vi "Turn.vi"(5 "角度":dbl format="%#_13g", 11 "error in (no error)":errorcluster) -> (15 "error out":errorcluster)   [LabVIEW 2019]
panel:
  out "馬達電壓":dbl[][](graph)
  out "SPD":dbl[](graph)
  out "POS":dbl[](graph)
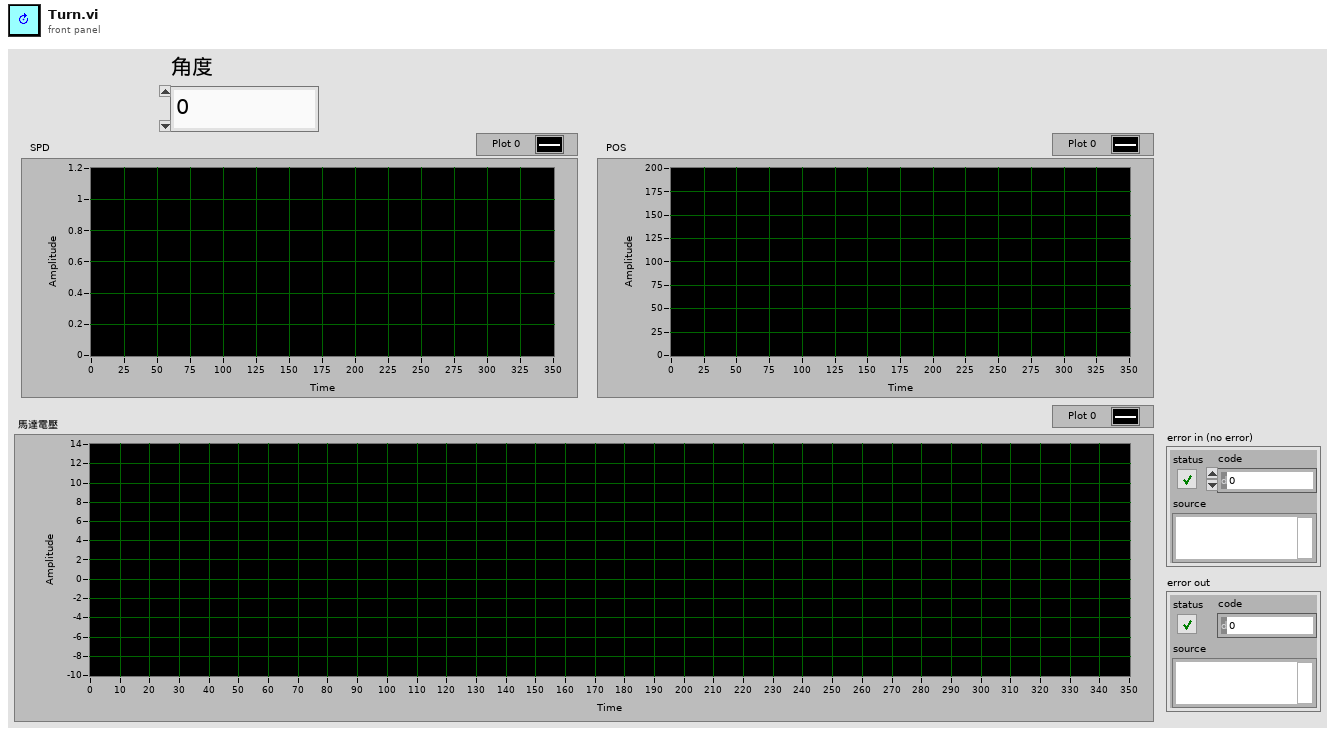
[diagram p1: front panel]
types:
  T1 = cluster{"proportional gain (Kc)":dbl, "integral time (Ti, min)":dbl, "derivative time (Td, min)":dbl}
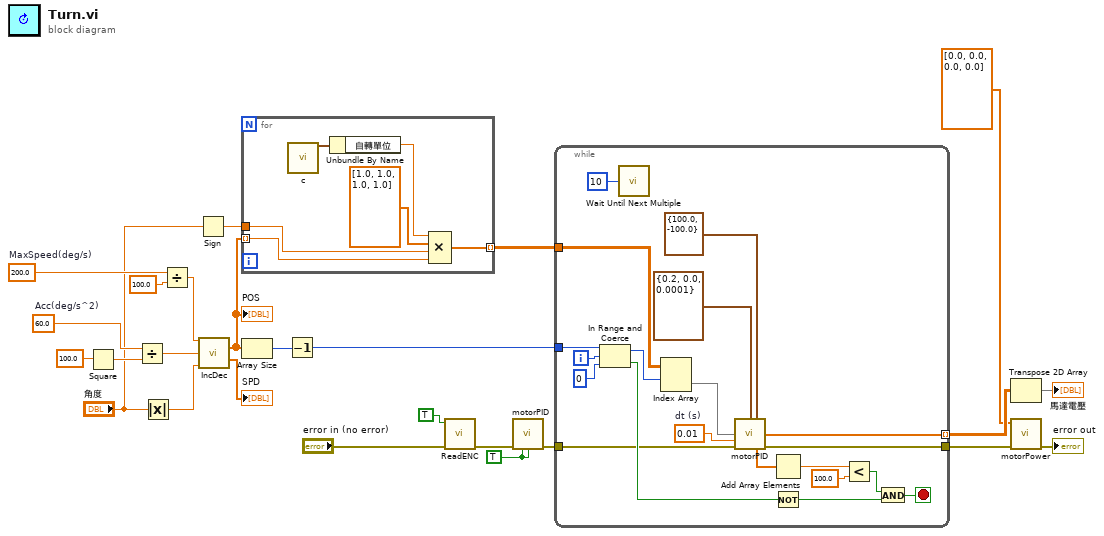
[diagram p0: block diagram]
diagram:
  w7 = 60.0  # Acc(deg/s^2)
  w4 = 200.0  # MaxSpeed(deg/s)
  w19 = TRUE ("reinitialize? (F)")
  n1 = Square(x=100.0 ("y")) -> (x^2=w14:dbl)
  n2 = Divide(x=w7, y=w14) -> (x/y=w15:dbl)
  n3 = Absolute Value(x="角度") -> (abs(x)=w11:dbl)
  n4 = Divide(x=w4, y=100.0) -> (x/y=w10:dbl)
  n5 = Sign(1:"角度") -> (0:w9:dbl)
  n6 = call "IncDec.vi"("MaxSpeed"=w10, "Acc"=w15, "Target"=w11) -> ("Position"=w12:dbl[], "Speed"=→"SPD":dbl[])  [unwired: 11 in]
  "POS" <- w12
  n7 = for {
    tunnel: w12 -> [w29] mode=indexing
    tunnel: [w31] -> w1 mode=indexing
    tunnel: w9 -> [w28]
    n8 = call "c.vi"() -> ("移動單位"=w27:cluster{"移動單位":dbl, "自轉單位":dbl})  [unwired: 15 in]
    n9 = Unbundle By Name(w27) -> ("自轉單位"=w30:dbl)
    n10 = Compound Arithmetic op=MULTIPLY(w30, dbl[] [1.0, 1.0, 1.0, 1.0] ("y"), w28, w29) -> (w31:dbl[])
  }
  n11 = Array Size(array=w12) -> (size(s)=w8:i32)
  n12 = Decrement(x=w8) -> (x-1=w2:i32)
  n13 = call "ReadENC.vi"("error in (no error)"="error in (no error)", "Reset"=TRUE) -> ("error out"=w18:errorcluster)  [unwired: 8 in, 1 out]
  n14 = call "motorPID.vi"("error in (no error)"=w18, "reinitialize? (F)"=w19, "EncRst"=w19) -> ("error out"=w20:errorcluster)  [unwired: 9 in, 3 out]
  n15 = while {
    tunnel: [w37] -> w25 mode=indexing
    tunnel: w20 -> [w35]
    tunnel: [w34] -> w22
    tunnel: w2 -> [w33]
    tunnel: w1 -> [w32]
    i -> [w43]
    stop <- w42 stop-if-true
    w38 = 0.01  # dt (s)
    n16 = In Range and Coerce(upper limit=w33, x=w43, lower limit=0) -> (coerced(x)=w47:i32, In Range?=w46:bool)
    n17 = call "Wait Until Next Multiple"("Count(mSec)"=u32 10) -> ()  [unwired: 1 out]
    n18 = Index Array(array=w32, index (row)=w47) -> (element=w39:dbl[])  [unwired: 1 in]
    n19 = call "motorPID.vi"("PID gains"=T1 {"proportional gain (Kc)"=0.2, "integral time (Ti, min)"=0.0, "derivative time (Td, min)"=0.0001}, "output range"=cluster{"output high":dbl, "output low":dbl} {"output high"=100.0, "output low"=-100.0}, "目標"=w39, "dt (s)"=w38, "error in (no error)"=w35) -> ("power"=w37:dbl[], "差值"=w36:dbl[], "error out"=w34:errorcluster)  [unwired: 7 in, 1 out]
    n20 = Add Array Elements(numeric array=w36) -> (sum=w50:dbl)
    n21 = Not(x=w46) -> (.not. x?=w44:bool)
    n22 = Less?(x=w50, y=100.0) -> (x < y?=w45:bool)
    n23 = And(x=w45, y=w44) -> (x .and. y?=w42:bool)
  }
  n24 = Transpose 2D Array(2D array=w25) -> (transposed array=→"馬達電壓":dbl[][])
  n25 = call "motorPower.vi"("error in (no error)"=w22, "DC_Pwr"=dbl[] [0.0, 0.0, 0.0, 0.0]) -> ("error out"=→"error out":errorcluster)  [unwired: 9 in]
